vi "LabVIEWpostman.vi"() -> ()   [LabVIEW 2015]
uses:
  <vilib>/httpClient/LabVIEWHTTPClient.lvlib
panel:
  in  "Properties in Service":string[][](array[string])=[["Temperature", "2"], ["Photocell", "7"], ["Button", "false"], ["Potentiometer", "10"], ["", ""], ["", ""], ["", ""], ["", ""], ["", ""], ["", ""], ["", ""]]
  in  "Service Name":string="UpdateValues"
  out "Properties":string[][](array[string])
  out "ThingWorx Response":string
  in  "Beginning of Url":string="http://52.202.159.58:80/Thingworx/Things/GenericEdge"
  in  "app key":string="?appKey=0aae8b5f-871a-4973-bdf2-199fabb27dcb"
  in  "Value of Property":string
  in  "Property":string
  out "error out":errorcluster
  in  "Type of Request":u16(ring)=1 items=["Put", "Post", "Get"]
  # "Get"
  # "All"
  # "Put"
  # "All"
  # "Post"
  # "*note: if you want to set a \nboolean to false or true, \nset the property value to \n0 or 1 respectively"
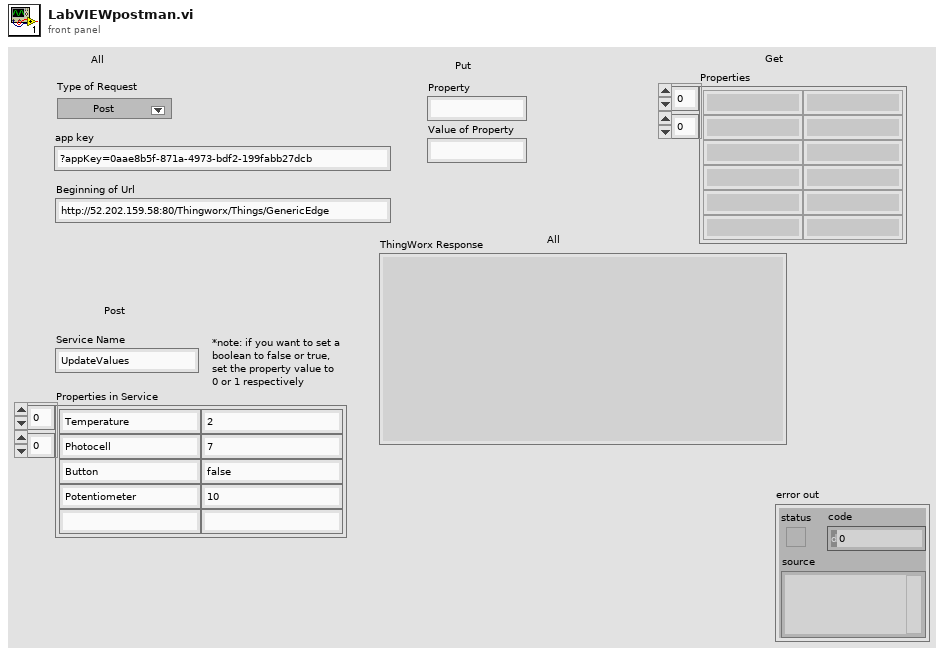
[diagram p1: front panel]
types:
  T1 = typedef "LabVIEWHTTPClient.lvlib/ClientHandle.ctl" = refnum<k1>
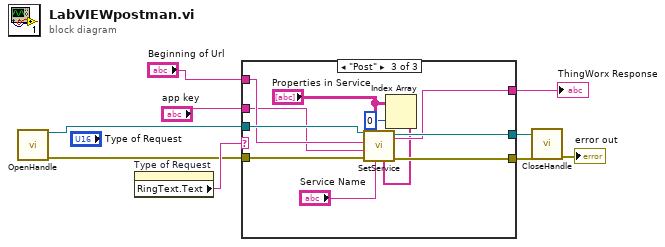
[diagram p0: block diagram]
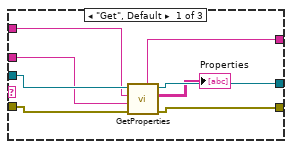
[diagram p2: hidden frame]
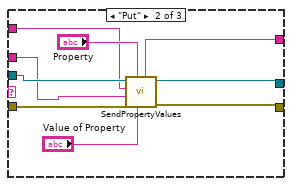
[diagram p3: hidden frame]
diagram:
  n1 = call <vilib>:"OpenHandle.vi"() -> ("client handle out"=w8:T1, "error out"=w7:errorcluster)  [unwired: 14 in]
  n2 = property on="Type of Request" class="Ring (strict)"() -> ("RingText.Text"=w9:string)  [unwired: 2 in, 2 out]
  n3 = case shown="\"Post\"" w9 {
    tunnel: w8 -> [w17 w26 w37]
    tunnel: w7 -> [w15 w25 w36]
    tunnel: [w16 w23 w35] -> w6
    tunnel: [w14 w24 w34] -> w5
    tunnel: [w13 w18 w33] -> w1
    tunnel: "app key" -> [w10 w20 w31]
    tunnel: "Beginning of Url" -> [w11 w19 w32]
    frame "Get", Default {
      n4 = call "GetProperties.vi"("error in (no error)"=w15, "appKey"=w10, "url beginning"=w11, "client handle"=w17) -> ("error out"=w14:errorcluster, "Array"=→"Properties":string[][], "client handle out"=w16:T1, "ThingWorx Response"=w13:string)  [unwired: 3 in, 1 out]
    }
    frame "Put" {
      n5 = call "SendPropertyValues.vi"("Value of Property"="Value of Property", "Property"="Property", "error in (no error)"=w25, "appKey"=w20, "Beginning of Url"=w19, "Refnum in"=w26) -> ("error out"=w24:errorcluster, "Refnum out"=w23:T1, "body"=w18:string)  [unwired: 1 in, 2 out]
    }
    frame "Post" {
      n6 = Index Array(array="Properties in Service", index (col)=0 ("disabled index (col)")) -> (element=w27:string[])  [unwired: 1 in]
      n7 = call "SetService.vi"("Properties in Service"=w27, "Service Name"="Service Name", "Properties"="Properties in Service", "error in"=w36, "appKey"=w31, "uri beginning"=w32, "client handle"=w37) -> ("error out"=w34:errorcluster, "client handle out"=w35:T1, "body"=w33:string)  [unwired: 2 out]
    }
  }
  "ThingWorx Response" <- w1
  n8 = call <vilib>:"CloseHandle.vi"("client handle"=w6, "error in (no error)"=w5) -> ("error out"=→"error out":errorcluster)  [unwired: 13 in]
